vi "Load Last Sync From File.vi"(8 "error in (no error)":errorcluster, 11 "Data Manager in":refnum<class "Data Manager.lvclass">) -> (0 "error out":errorcluster, 3 "Data Manager out":refnum<class "Data Manager.lvclass">)   [LabVIEW 2020, in "Data Manager.lvclass"]
uses:
  Data Manager.lvclass
  Data Manager.lvclass/Data Manager.ctl
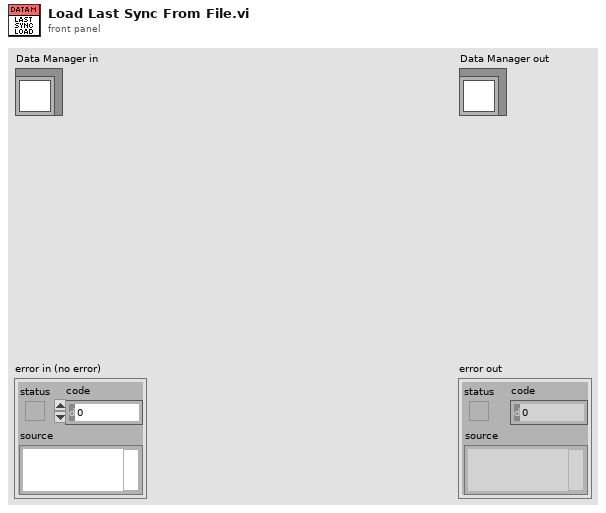
[diagram p1: front panel]
types:
  T1 = typedef "Data Manager.lvclass/Strava JSON for Club Activities--cluster.ctl" = cluster{"athlete":cluster{"firstname":string, "lastname":string}, "type":string, "distance":dbl, "moving_time":dbl, "elapsed_time":dbl, "total_elevation_gain":dbl}
  T2 = typedef "Data Manager.lvclass/Name--cluster.ctl" = cluster{"First":string, "Last":string}
  T3 = typedef "Data Manager.lvclass/Profile--cluster.ctl" = cluster{"Alias":string, "Team":string}
  T4 = cluster{"Strava JSON Last Sync":T1, "Athlete Profile Map":map{T2, T3}}
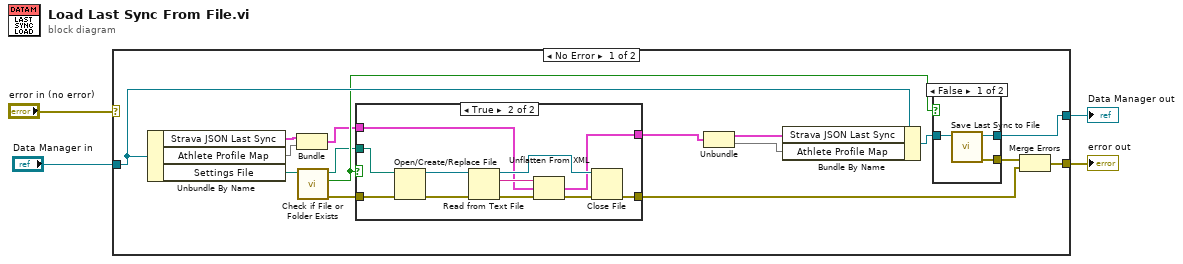
[diagram p0: block diagram]
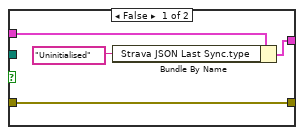
[diagram p2: hidden frame]
diagram:
  n1 = case shown="No Error" "error in (no error)" {
    selector: "error in (no error)" -> [_ w41]
    tunnel: [w19 w41] -> w3
    tunnel: [w17 w40] -> w1
    tunnel: "Data Manager in" -> [w20 w40]
    frame No Error {
      n2 = Unbundle By Name(w20) -> ("Strava JSON Last Sync"=w10:T1, "Athlete Profile Map"=w9:map{T2, T3}, "Settings File"=w11:path)
      n3 = Bundle("Strava JSON Last Sync"=w10, "Athlete Profile Map"=w9) -> (w8:T4)  [unwired: 1 in]
      n4 = call <vilib>:"Check if File or Folder Exists.vi"("path"=w11) -> ("error out"=w13:errorcluster, "file or folder exists?"=w15:bool, "dup path"=w14:path)  [unwired: 8 in]
      n5 = case shown="True" w15 {
        tunnel: w14 -> [_ w35]
        tunnel: w8 -> [w24 w28]
        tunnel: [w23 w27] -> w7
        tunnel: w13 -> [w21 w31]
        tunnel: [w21 w30] -> w12
        frame False {
          n6 = Bundle By Name(cluster=w24, "Strava JSON Last Sync.type"="Uninitialised" ("type")) -> (w23:T4)
        }
        frame True {
          n7 = Open/Create/Replace File(file path (use dialog)=w35, error in=w31) -> (refnum out=w34:refnum<file>, error out=w32:errorcluster)  [unwired: 4 in, 1 out]
          n8 = Read from Text File(file (use dialog)=w34, error in=w32) -> (refnum out=w33:refnum<file>, text=w29:string, error out=w25:errorcluster)  [unwired: 2 in, 1 out]
          n9 = Unflatten From XML(xml string=w29, type=w28, error in (no error)=w25) -> (value=w27:T4, error out=w26:errorcluster)
          n10 = Close File(refnum=w33, error in=w26) -> (error out=w30:errorcluster)  [unwired: 1 out]
        }
      }
      n11 = Unbundle(w7) -> ("Strava JSON Last Sync"=w6:T1, "Athlete Profile Map"=w5:map{T2, T3})
      n12 = Bundle By Name(cluster=w20, "Strava JSON Last Sync"=w6, "Athlete Profile Map"=w5) -> (w18:refnum<class "Data Manager.lvclass">)
      n13 = case shown="False" w15 {
        tunnel: w18 -> [w38 w39]
        tunnel: [w37 w39] -> w17
        tunnel: [w36 _] -> w16
        frame False {
          n14 = call-dynamic "Save Last Sync to File.vi"("Data Manager in"=w38) -> ("error out"=w36:errorcluster, "Data Manager out"=w37:refnum<class "Data Manager.lvclass">)  [unwired: 9 in]
        }
        frame True {
        }
      }
      n15 = Merge Errors(w16, w12) -> (w19:errorcluster)
    }
    frame Error {
    }
  }
  "error out" <- w3
  "Data Manager out" <- w1
